vi "2013_01_17 remove DC offset.vi"(11 "Waveform in":waveform(dbl)) -> (3 "Waveform out":waveform(dbl))   [LabVIEW 2013]
uses:
  <vilib>/measure/madcrms.llb/Averaged DC-RMS for 1 Chan.vi
  <vilib>/measure/NI_MAPro.lvlib
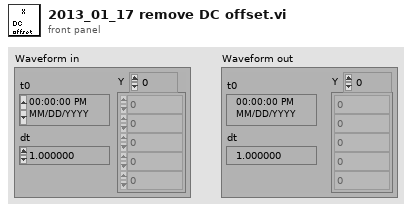
[diagram p1: front panel]
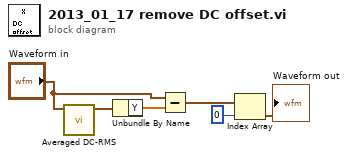
[diagram p0: block diagram]
diagram:
  n1 = call-poly <vilib>:"Averaged DC-RMS.vi"("signal in"="Waveform in") -> ("DC value waveform"=w1:waveform(dbl))  [unwired: 6 in, 4 out]
  n2 = Unbundle By Name(w1) -> ("Y"=w2:dbl[])
  n3 = Subtract(x="Waveform in", y=w2) -> (x-y=w4:waveform(dbl)[])
  n4 = Index Array(array=w4, index=0) -> (element=→"Waveform out":waveform(dbl))
